vi "1D_Array_Average.vi"(11 "Array In":dbl[](array[numeric])) -> (2 "Array Size":i32, 3 "Array Average":dbl)   [LabVIEW 2014]
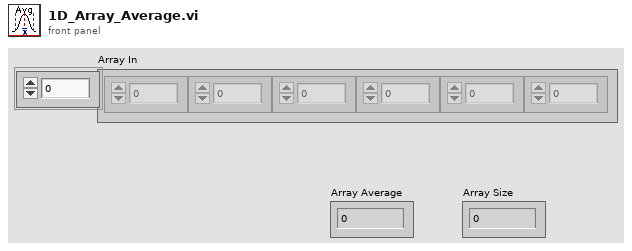
[diagram p1: front panel]
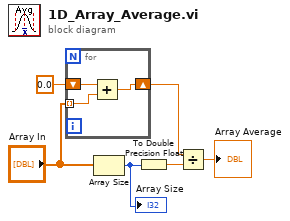
[diagram p0: block diagram]
diagram:
  n1 = for {
    tunnel: "Array In" -> [w8] mode=indexing
    shift-right: [w9] -> w5
    shift-left: 0.0 ("Numeric Control") -> [w7]
    n2 = Add(x=w7, y=w8) -> (x+y=w9:dbl)
  }
  n3 = Array Size(array="Array In") -> (size(s)=w1:i32)
  "Array Size" <- w1
  n4 = To Double Precision Float(number=w1) -> (double precision float=w2:dbl)
  n5 = Divide(x=w5, y=w2) -> (x/y=→"Array Average":dbl)
